vi "Destroy Message Transport.vi"(8 "error in":errorcluster, 11 "NotifierMessageTransport in":refnum<class "NotifierMessageTransport.lvclass">) -> (0 "error out":errorcluster, 3 "NotifierMessageTransport out":refnum<class "NotifierMessageTransport.lvclass">)   [LabVIEW 2016, in "NotifierMessageTransport.lvclass"]
uses:
  NotifierMessageTransport.lvclass
panel:
  # "INPUTS"
  # "OUTPUTS"
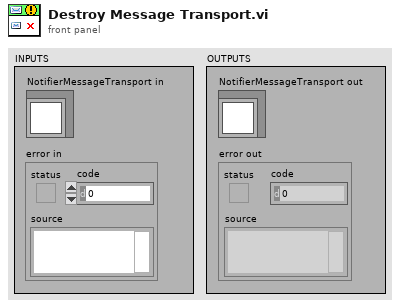
[diagram p1: front panel]
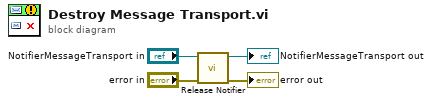
[diagram p0: block diagram]
diagram:
  n1 = call "Release Notifier.vi"("error in"="error in", "NotifierMessageTransport in"="NotifierMessageTransport in") -> ("error out"=→"error out":errorcluster, "NotifierMessageTransport out"=→"NotifierMessageTransport out":refnum<class "NotifierMessageTransport.lvclass">)  [unwired: 8 in]
